vi "Configure Wiring.vi"(0 "VISA resource name":refnum<visa-resource-name>, 3 "Wiring A (1: 1p2W)":i32(ring)=1 items=["1P2W"=1, "1P3W"=2, "3P3W"=3, "3P4W"=4, "3V3A"=5], 11 "error in (no error)":errorcluster) -> (4 "VISA resource name out":refnum<visa-resource-name>, 15 "error out":errorcluster)   [LabVIEW 2016, in "Yokogawa WT300 Series.lvlib"]
doc: "Sets the wiring system."
uses:
  Yokogawa WT300 Series.lvlib
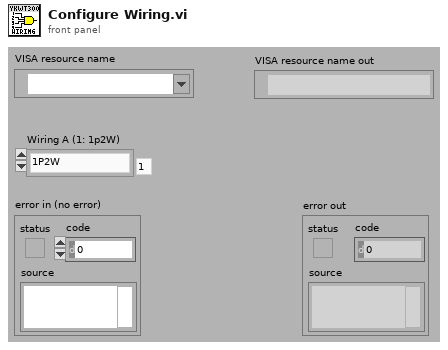
[diagram p1: front panel]
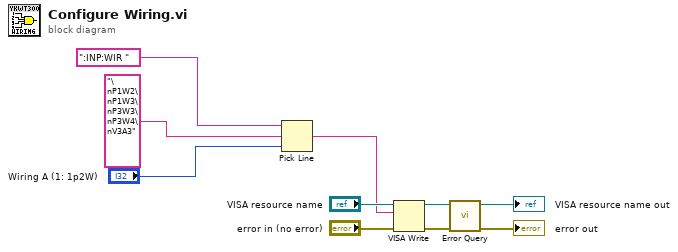
[diagram p0: block diagram]
diagram:
  n1 = Pick Line ("ライン選択")(string ("")=":INP:WIR ", multi-line string="\nP1W2\nP1W3\nP3W3\nP3W4\nV3A3", line index="Wiring A (1: 1p2W)") -> (output string=w4:string)
  n2 = VISA Write ("VISA書き込み")(VISA resource name="VISA resource name", write buffer=w4, error in (no error)="error in (no error)") -> (VISA resource name out=w6:refnum<visa-resource-name>, error out=w5:errorcluster)  [unwired: 1 out]
  n3 = call "Error Query.vi"("error in (no error)"=w5, "VISA resource name"=w6) -> ("error out"=→"error out":errorcluster, "VISA resource name out"=→"VISA resource name out":refnum<visa-resource-name>)  [unwired: 6 in, 2 out]
